vi "_Main_LookOnly_V1.1.vi"() -> ()   [LabVIEW 2017]
uses:
  <vilib>/Instr/_visa.llb/VISA Configure Serial Port (Instr).vi
panel:
  in  "DAC 1 LIMIT, V":dbl min=-50.0 max=50.0 format="%#_5g"
  in  "DAC 2, V":dbl min=-10.0 max=10.0 format="%#_5g"
  in  "DAC 1, V":dbl min=-50.0 max=50.0 format="%#_5g"
  out "DAC1volt, V":dbl
  out "Field LOG":cluster{dbl[], dbl[]}(graph)
  out "LED2":bool
  out "LED1":bool
  out "Bytes at Port":u32
  out "RecTry":i32
  out "Field, kV/cm":dbl
  out "VoltageRes, V":dbl
  out "PlotPoints":cluster{"Time":dbl[], "Voltage":dbl[]}(graph)={"Time"=[0.0, 0.00037111111108161925, 0.000510833333311085, 0.0006505555555405509, 0.0007766666666915019, 0.0009172222221968695, 0.0010569444444263353, 0.0011958333333152243, 0.0013350000000274223], "Voltage"=[5.89, 5.89, 5.89, 5.89, 5.89, 5.89, 5.89, 5.89, 5.89]}
  out "VoltageBelow, V":dbl
  out "Knob":u32
  out "Current, mA":dbl format="%#_4g"
  out "Channel 4, V":dbl format="%#_5g"
  out "Channel 3, V":dbl format="%#_5g"
  out "Channel 2, V":dbl format="%#_5g"
  out "Channel 1, V":dbl format="%#_5g"
  in  "Stop Button":bool
  in  "Start Button":bool
  in  "film H, nm":dbl=50.0
  in  "6 electrodes":bool
  out "Shutter Red":bool
  out "Shutter Green":bool
  in  "COM port":refnum<visa-resource-name>
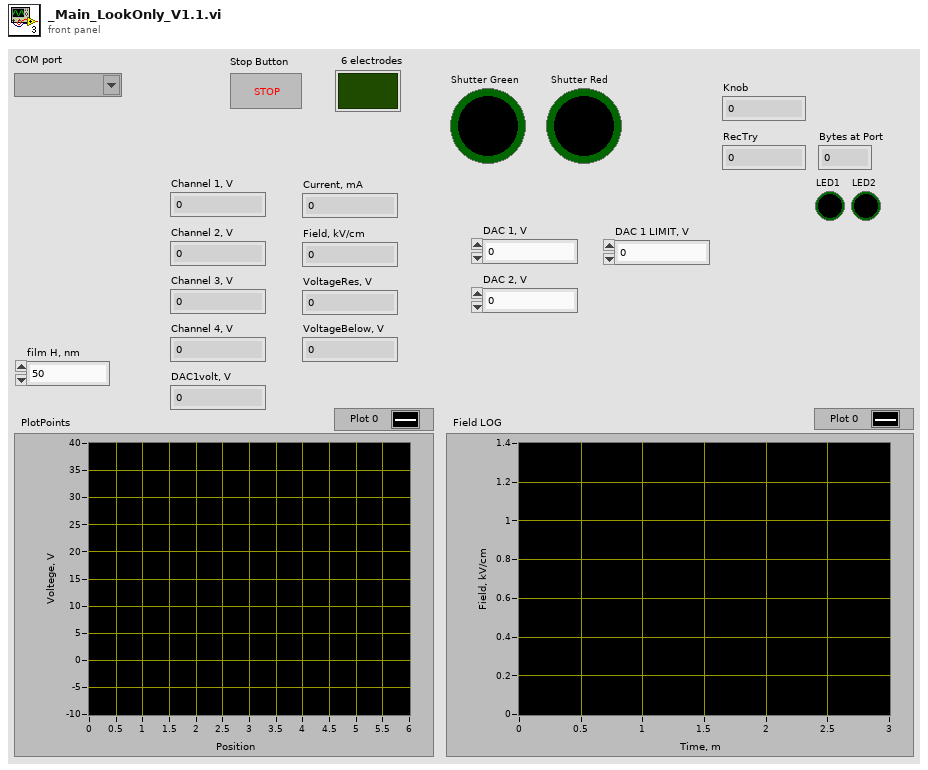
[diagram p1: front panel]
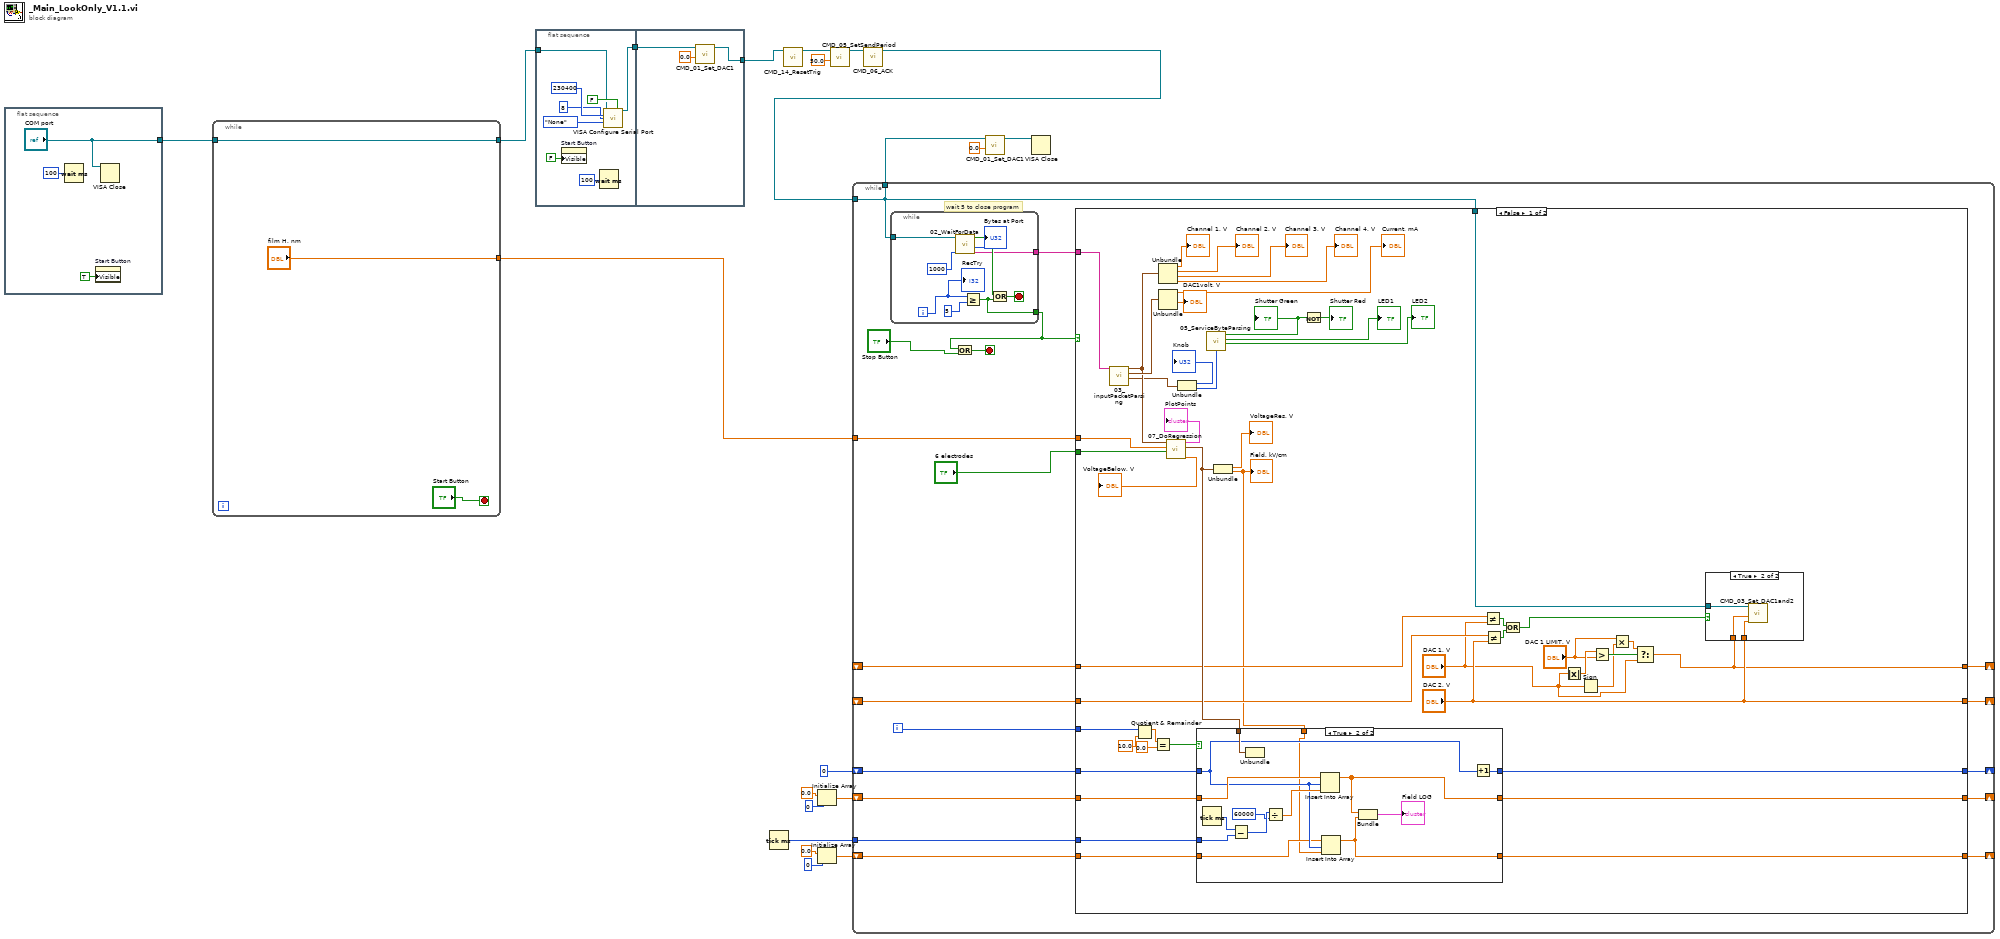
[diagram p0: block diagram]
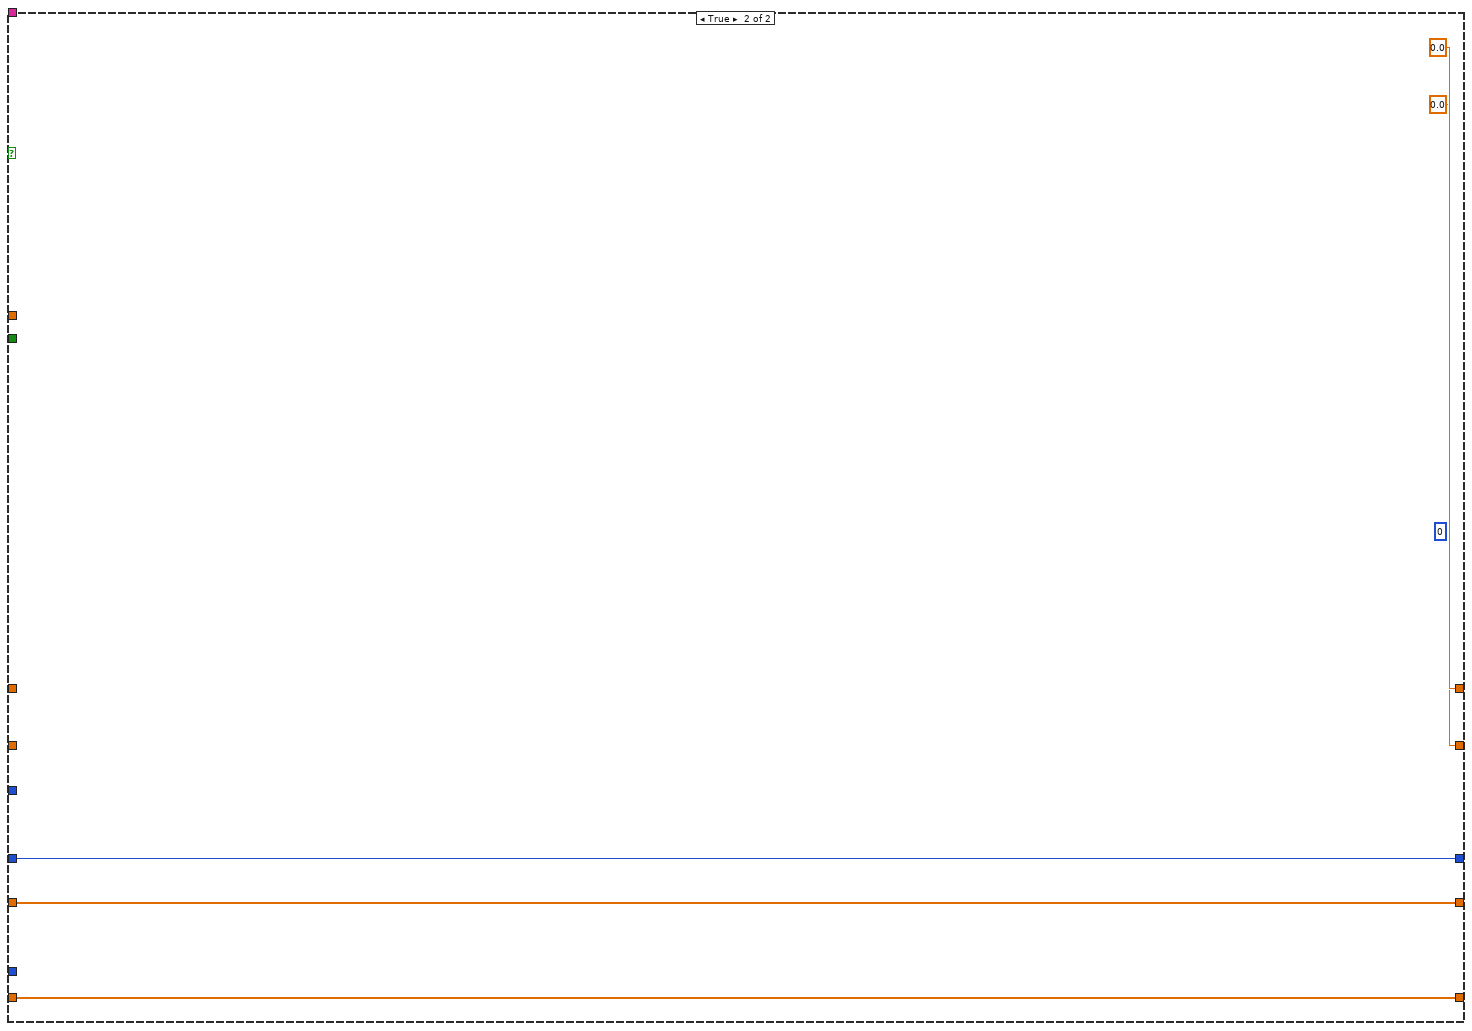
[diagram p4: hidden frame]
diagram:
  n1 = flat-sequence {
    tunnel: ["COM port"] -> w20
    frame #0 {
      n2 = Wait (ms)(milliseconds to wait=u32 100) -> ()  [unwired: 1 out]
      n3 = property on="Start Button" class="Bool"("Visible"=TRUE) -> ()  [unwired: 2 in, 2 out]
      n4 = VISA Close(VISA resource name="COM port") -> ()  [unwired: 1 in, 1 out]
    }
  }
  n5 = while {
    tunnel: w20 -> [w25]
    tunnel: [w25] -> w19
    tunnel: ["film H, nm"] -> w18
    stop <- "Start Button" stop-if-true
  }
  n6 = flat-sequence {
    tunnel: w19 -> [w30]
    tunnel: [w29] -> w9
    tunnel: [w37] -> w16
    tunnel: w9 -> [w36]
    frame #0 {
      n7 = property on="Start Button" class="Bool"("Visible"=FALSE) -> ()  [unwired: 2 in, 2 out]
      n8 = Wait (ms)(milliseconds to wait=u32 100) -> ()  [unwired: 1 out]
      n9 = call-poly "VISA Configure Serial Port"("VISA resource name"=w30, "Enable Termination\nChar (T)"=FALSE ("Enable Termination\nChar (T)"), "baud rate (9600)"=u32 230400, "data bits (8)"=u16 8, "parity (0:none)"=enum16{"None", "Odd", "Even", "Mark", "Space"}."None") -> ("VISA resource name out"=w29:refnum<visa-resource-name>)  [unwired: 9 in, 1 out]
    }
    frame #1 {
      n10 = call "CMD_01_Set_DAC1.vi"("Input, V"=0.0, "VISA resource name"=w36) -> ("VISA resource name out"=w37:refnum<visa-resource-name>)  [unwired: 9 in]
    }
  }
  n11 = Tick Count (ms)() -> (millisecond timer value=w4:u32)
  n12 = call "CMD_14_ResetTrig.vi"("VISA resource name"=w16) -> ("VISA resource name out"=w12:refnum<visa-resource-name>)  [unwired: 10 in]
  n13 = Initialize Array(0.0 ("element"), 0 ("dimension size")) -> (w1:dbl[])
  n14 = Initialize Array(0.0 ("element"), 0 ("dimension size")) -> (w5:dbl[])
  n15 = call "CMD_05_SetSendPeriod.vi"("Period, ms"=50.0, "VISA resource name"=w12) -> ("VISA resource name out"=w11:refnum<visa-resource-name>)  [unwired: 9 in]
  n16 = call "CMD_06_ACK.vi"("VISA resource name"=w11) -> ("VISA resource name out"=w10:refnum<visa-resource-name>)  [unwired: 10 in]
  n17 = while {
    tunnel: w10 -> [w51]
    tunnel: [w51] -> w17
    tunnel: w18 -> [w53]
    shift-right: [w49] -> _
    shift-left: 0 -> [w50]
    tunnel: w4 -> [w47]
    shift-right: [w45] -> _
    shift-left: w5 -> [w48]
    shift-right: [w44] -> _
    shift-left: w1 -> [w46]
    shift-right: [w42] -> _
    shift-left: _ -> [w39]
    shift-right: [w41] -> _
    shift-left: _ -> [w40]
    i -> [w52]
    stop <- w56 stop-if-true
    # "wait 5 to close program"
    n18 = while {
      tunnel: w51 -> [w131]
      tunnel: [w134] -> w55
      tunnel: [w135] -> w54
      i -> [w133]
      stop <- w137 stop-if-true
      n19 = call "02_WaitForData.vi"("WaitTimeoutMS"=u32 1000, "VISA"=w131) -> ("Buffer"=w135:string, "Bytes at Port"=→"Bytes at Port":u32, "Data Recived"=w136:bool)  [unwired: 7 in]
      n20 = Greater Or Equal?(x=w133, y=5) -> (x >= y?=w134:bool)
      n21 = Or(x=w136, y=w134) -> (x .or. y?=w137:bool)
      "RecTry" <- w133
    }
    n22 = Or(x=w55, y="Stop Button") -> (x .or. y?=w56:bool)
    n23 = case shown="False" w55 {
      tunnel: w54 -> [w105 _]
      tunnel: w53 -> [w94 _]
      tunnel: "6 electrodes" -> [w93 _]
      tunnel: w52 -> [w83 _]
      tunnel: w51 -> [w65 _]
      tunnel: w50 -> [w81 w130]
      tunnel: [w80 w130] -> w49
      tunnel: w48 -> [w78 w129]
      tunnel: w47 -> [w77 _]
      tunnel: w46 -> [w76 w128]
      tunnel: [w74 w129] -> w45
      tunnel: [w73 w128] -> w44
      tunnel: [w59 0.0 ("DAC 1, V")] -> w42
      tunnel: ["DAC 2, V" 0.0 ("DAC 2, V")] -> w41
      tunnel: w40 -> [w69 _]
      tunnel: w39 -> [w68 _]
      frame False {
        n24 = call "03_inputPacketParsing.vi"("string"=w105) -> ("Service state"=w91:cluster{u8, u8}, "DAC state"=w100:cluster{dbl, dbl, dbl, dbl}, "Voltage"=w92:cluster{dbl, dbl, dbl, dbl})  [unwired: 6 in, 2 out]
        n25 = Quotient & Remainder(x=w83, y=10.0) -> (x-y*floor(x/y)=w86:dbl)  [unwired: 1 out]
        n26 = Equal?(x=w86, y=0.0) -> (x = y?=w82:bool)
        n27 = Unbundle(w92) -> (→"Channel 1, V":dbl, →"Channel 2, V":dbl, →"Channel 3, V":dbl, →"Channel 4, V":dbl)
        n28 = Unbundle(w100) -> (→"Current, mA":dbl, →"DAC1volt, V":dbl)  [unwired: 2 out]
        n29 = call "07_DoRegression.vi"("6 electrodes"=w93, "film H, nm"=w94, "Input ChVoltage"=w92) -> ("VoltageBelow, V"=→"VoltageBelow, V":dbl, "Regression"=w79:cluster{"VoltageRes, V":dbl, "Field, kV/cm":dbl}, "PlotPoints"=→"PlotPoints":cluster{"Time":dbl[], "Voltage":dbl[]})  [unwired: 6 in]
        n30 = Unbundle(w91) -> (→"Knob":u8, w90:u8)
        n31 = call "05_ServiceByteParsing.vi"("InputByte"=w90) -> ("LED2"=→"LED2":bool, "LED1"=→"LED1":bool, "TrigState"=w89:bool)  [unwired: 7 in, 1 out]
        "Shutter Green" <- w89
        n32 = Unbundle(w79) -> ("VoltageRes, V"=→"VoltageRes, V":dbl, "Field, kV/cm"=w57:dbl)
        "Field, kV/cm" <- w57
        n33 = case shown="True" w82 {
          tunnel: w81 -> [w111 w117]
          tunnel: [w111 w120] -> w80
          tunnel: w79 -> [_ w125]
          tunnel: w78 -> [w109 w118]
          tunnel: w77 -> [_ w123]
          tunnel: w76 -> [w110 w116]
          tunnel: [w110 w114] -> w73
          tunnel: [w109 w113] -> w74
          tunnel: w57 -> [_ w112]
          frame False {
          }
          frame True {
            n34 = Tick Count (ms)() -> (millisecond timer value=w124:u32)
            n35 = Subtract(x=w124, y=w123) -> (x-y=w122:u32)
            n36 = Unbundle(w125) -> ()  [unwired: 2 out]
            n37 = Divide(x=w122, y=u32 60000) -> (x/y=w119:dbl)
            n38 = Insert Into Array(array=w118, index=w117, new element=w119) -> (w113:dbl[])
            n39 = Insert Into Array(array=w116, index=w117, new element=w112) -> (w114:dbl[])
            n40 = Bundle(w113, w114) -> (→"Field LOG":cluster{dbl[], dbl[]})  [unwired: 1 in]
            n41 = Increment(x=w117) -> (x+1=w120:i32)
          }
        }
        n42 = Not(x=w89) -> (.not. x?=→"Shutter Red":bool)
        n43 = Not Equal?(x=w68, y="DAC 1, V") -> (x != y?=w71:bool)
        n44 = Not Equal?(x=w69, y="DAC 2, V") -> (x != y?=w70:bool)
        n45 = Or(x=w71, y=w70) -> (x .or. y?=w67:bool)
        n46 = Absolute Value(x="DAC 1, V") -> (abs(x)=w64:dbl)
        n47 = Sign(1:"DAC 1, V") -> (0:w61:dbl)
        n48 = Greater?(x=w64, y="DAC 1 LIMIT, V") -> (0:w63:bool)
        n49 = Multiply(x="DAC 1 LIMIT, V", y=w61) -> (x*y=w62:dbl)
        n50 = Select(t=w62, s=w63, f="DAC 1, V") -> (s? t:f=w59:dbl)
        n51 = case shown="True" w67 {
          tunnel: "DAC 2, V" -> [_ w108]
          tunnel: w59 -> [_ w107]
          tunnel: w65 -> [_ w106]
          frame False {
          }
          frame True {
            n52 = call "CMD_03_Set_DAC1and2.vi"("Input2, V"=w108, "Input1, V"=w107, "VISA resource name"=w106) -> ()  [unwired: 8 in, 1 out]
          }
        }
      }
      frame True {
        (unwired) u32 0
      }
    }
  }
  n53 = call "CMD_01_Set_DAC1.vi"("Input, V"=0.0, "VISA resource name"=w17) -> ("VISA resource name out"=w14:refnum<visa-resource-name>)  [unwired: 9 in]
  n54 = VISA Close(VISA resource name=w14) -> ()  [unwired: 1 in, 1 out]
